vi "Conv_Meters_Inches.vi"(10 "Meters":dbl) -> (2 "Inches":dbl)   [LabVIEW 2019, in "Trajectory_Library.lvlib"]
doc: "Convert Meters to Inches"
uses:
  Trajectory_Library.lvlib
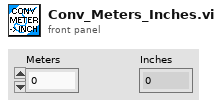
[diagram p1: front panel]
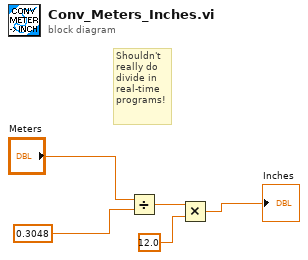
[diagram p0: block diagram]
diagram:
  # "Shouldn't\nreally do\ndivide in\nreal-time\nprograms!"
  n1 = Divide(x="Meters", y=0.3048) -> (x/y=w3:dbl)
  n2 = Multiply(x=w3, y=12.0) -> (x*y=→"Inches":dbl)
